vi "Slit.v.Full.vi"(2 "Under Scan /ms":dbl, 3 "Slit Delay":dbl, 4 "Scanning Mode":dbl, 5 "Camera Delay /ms":dbl) -> (0 "Prexposure /ms":dbl, 1 "Underscan /ms":dbl)   [LabVIEW 2016]
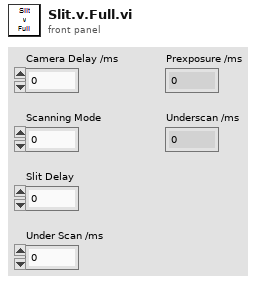
[diagram p1: front panel]
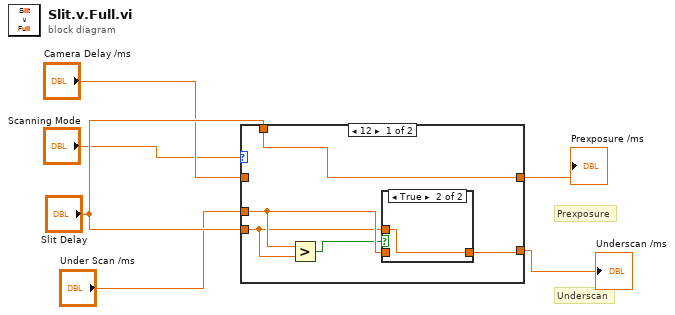
[diagram p0: block diagram]
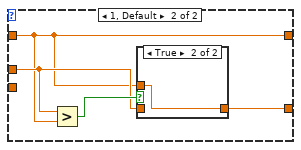
[diagram p3: hidden frame]
diagram:
  # "Prexposure"
  # "Underscan"
  n1 = case shown="12" "Scanning Mode" {
    tunnel: "Camera Delay /ms" -> [_ w14]
    tunnel: [w11 w14] -> w5
    tunnel: "Slit Delay" -> [w11 _]
    tunnel: "Under Scan /ms" -> [w9 w15]
    tunnel: "Slit Delay" -> [w8 _]
    tunnel: [w10 w17] -> w6
    frame 12 {
      n2 = Greater?(x=w9, y=w8) -> (0:w7:bool)
      n3 = case shown="True" w7 {
        tunnel: w9 -> [w12 _]
        tunnel: [w12 w13] -> w10
        tunnel: w8 -> [_ w13]
        frame False {
        }
        frame True {
        }
      }
    }
    frame 1, Default {
      n4 = Greater?(x=w15, y=w14) -> (0:w16:bool)
      n5 = case shown="True" w16 {
        tunnel: w15 -> [w18 _]
        tunnel: [w18 w19] -> w17
        tunnel: w14 -> [_ w19]
        frame False {
        }
        frame True {
        }
      }
    }
  }
  "Prexposure /ms" <- w5
  "Underscan /ms" <- w6
